vi "Write DMM DataSet.vi"(8 "error in (no error)":errorcluster, 10 "DMM DataSet":T1[](array[typedef]), 11 "DMM Instrument in":refnum<class "DMM Instrument.lvclass">) -> (0 "error out":errorcluster, 3 "DMM Instrument out":refnum<class "DMM Instrument.lvclass">)   [LabVIEW 2025]
uses:
  DMM Instrument.lvclass
  DMM Dataset.ctl
  DMM Instrument.lvclass/DMM Instrument.ctl
  C:/Users/Public/Documents/Sandia National Labs/TSS Plugin/Abstract PlugIn.lvlibp/Plugin/Abstract/Abstract Instrument/Abstract Instrument.lvclass
  C:/Users/Public/Documents/Sandia National Labs/TSS Plugin/CEF.lvlibp/serializable node/CEF_serializable node.lvclass
  C:/Users/Public/Documents/Sandia National Labs/TSS Plugin/CEF.lvlibp/Node/CEF_Node.lvclass
  C:/Working copy/tss/Plugin/DMM/DMM Instrument/DMM Instrument.lvclass
  C:/Users/Public/Documents/Sandia National Labs/TSS Plugin/Interface.lvlibp/Analog Input/AI.lvclass
  C:/Users/Public/Documents/Sandia National Labs/TSS Plugin/Interface.lvlibp/Digital Input/DI.lvclass
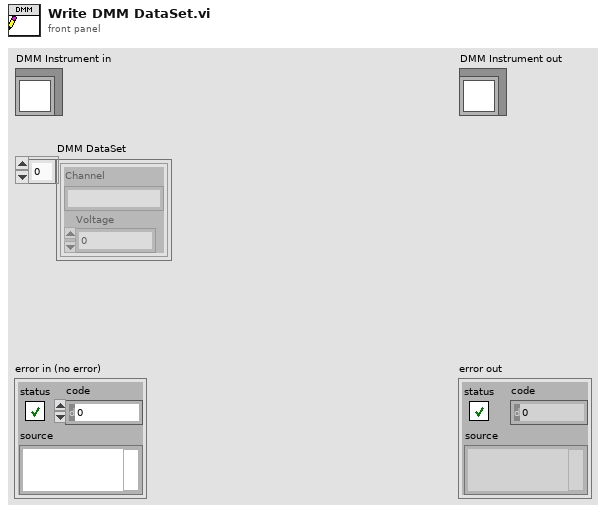
[diagram p1: front panel]
types:
  T1 = typedef "DMM Dataset.ctl" = cluster{"Channel":string, "Voltage":dbl}
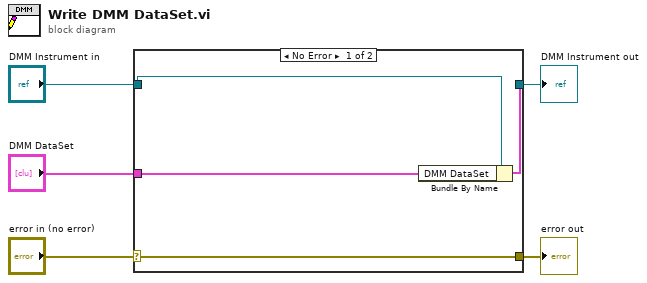
[diagram p0: block diagram]
diagram:
  n1 = case shown="No Error" "error in (no error)" {
    selector: "error in (no error)" -> [w9 w10]
    tunnel: [w9 w10] -> w4
    tunnel: [w7 w11] -> w2
    tunnel: "DMM Instrument in" -> [w8 w11]
    tunnel: "DMM DataSet" -> [w6 _]
    frame No Error {
      n2 = Bundle By Name(cluster=w8, "DMM DataSet"=w6) -> (w7:cluster{})
    }
    frame Error {
    }
  }
  "error out" <- w4
  "DMM Instrument out" <- w2
